vi "Test Test Case Status Correct When Collecting Method Result.vi"(8 "error in (no error)":errorcluster, 11 "Test Case In":refnum<class "Result Collector Tests.lvclass">) -> (0 "error out":errorcluster, 3 "Test Case Out":refnum<class "Result Collector Tests.lvclass">)   [LabVIEW 2020, in "Result Collector Tests.lvclass"]
uses:
  Result Collector Tests.lvclass
  C:/Program Files (x86)/National Instruments/LabVIEW 2020/vi.lib/Astemes/LUnit/Test Case.lvclass
  Framework/Result Collector/Result Collector.lvclass
  Result/Result.ctl
  Result/Status.ctl
  Result/Type.ctl
  Framework/Result Collector/Result Collector.lvclass/Result Collector.ctl
  <vilib>/Astemes/LUnit/Test Case.lvclass/Test Case.ctl
  7d523b10-b8d1-4baa-9334-5865d033fd32.vi
  Framework/Result Collector/Public/API/Collect Method Results.vi
  <vilib>/Astemes/LUnit/Palette/Pass.vi
  <vilib>/Astemes/LUnit/Palette/Fail.vi
  <vilib>/Astemes/LUnit/Compare Variants.vi
  <vilib>/Astemes/LUnit/Describe Comparison.vi
  <vilib>/Astemes/LUnit/Set Assertion Type.vi
  <vilib>/Astemes/LUnit/Add test result.vi
  <vilib>/Astemes/LUnit/Variant to string.vi
  <vilib>/Astemes/LUnit/LUnit Record Assertion Result.vi
  <vilib>/Astemes/LUnit/LUnit Aggregate Assertion Results.vi
  <vilib>/Astemes/LUnit/Method Result/LUnit Merge Status.vi
  <vilib>/Astemes/LUnit/LUnit Concatenate result strings.vi
  <vilib>/Utility/Data Type/Get Type Information.vi
  <vilib>/Utility/LVClass/Get LV Class Name.vi
  Result/Result.lvlib
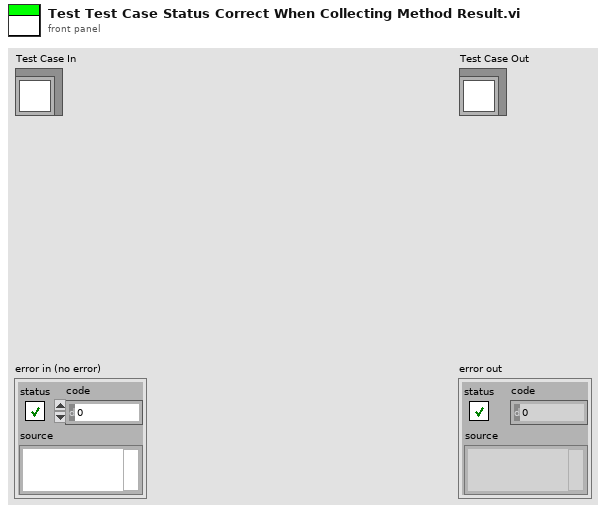
[diagram p1: front panel]
types:
  T1 = typedef "Result.lvlib/Status.ctl" = enum16{"Pass", "Fail", "Error", "Skipped", "Setup Error", "Broken", "Teardown Error"}
  T2 = typedef "Result.lvlib/Result.ctl" = cluster{"Case":string, "Method":string, "Message":string, "Description":string, "Status":T1, "Result Type":T3, "Execution Time":dbl}
  T3 = typedef "Result.lvlib/Type.ctl" = enum16{"Assertion", "Method", "Case", "Suite"}
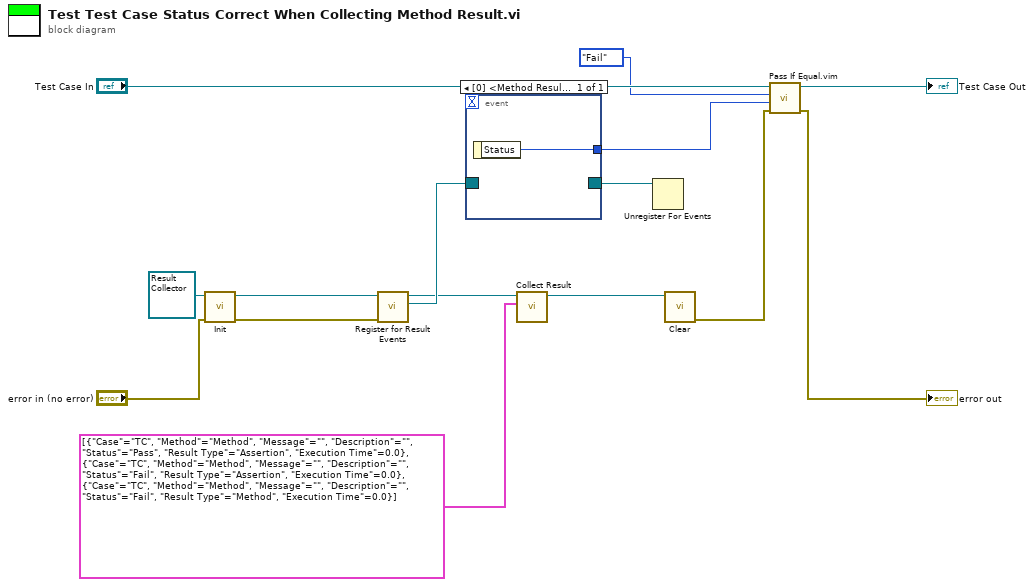
[diagram p0: block diagram]
diagram:
  n1 = call-dynamic "Init.vi"("error in (no error)"="error in (no error)", "Report Generator In"=refnum<class "Result Collector.lvclass"> refnum) -> ("error out"=w11:errorcluster, "Report Generator Out"=w12:refnum<class "Result Collector.lvclass">)  [unwired: 8 in]
  n2 = call "Register for Result Events.vi"("error in (no error)"=w11, "Result Collector In"=w12) -> ("Result Events"=w9:refnum<event-registration>, "Result Collector Out"=w7:refnum<class "Result Collector.lvclass">)  [unwired: 7 in, 1 out]
  n3 = event shown="[0] <Method Result>: User Event" {
    selector: w9 -> [_]
    dyn-events: [_] -> w8
    timeout: _ -> [_]
    tunnel: [w16] -> w4
    event User Event {
      n4 = event-data() -> ("Status"=w16:T1)  [unwired: 1 in]
    }
  }
  n5 = call "Collect Result.vi"("Results"=T2[] [{"Case"="TC", "Method"="Method", "Message"="", "Description"="", "Status"=enum."Pass", "Result Type"=enum."Assertion", "Execution Time"=0.0}, {"Case"="TC", "Method"="Method", "Message"="", "Description"="", "Status"=enum."Fail", "Result Type"=enum."Assertion", "Execution Time"=0.0}, {"Case"="TC", "Method"="Method", "Message"="", "Description"="", "Status"=enum."Fail", "Result Type"=enum."Method", "Execution Time"=0.0}], "Report Generator In"=w7) -> ("Report Generator Out"=w6:refnum<class "Result Collector.lvclass">)  [unwired: 9 in]
  n6 = Unregister For Events(event registration refnum=w8) -> ()  [unwired: 1 in, 1 out]
  n7 = call-dynamic "Clear.vi"("Report Generator In"=w6) -> ("error out"=w3:errorcluster)  [unwired: 9 in, 1 out]
  n8 = call "Pass If Equal.vim"("error in (no error)"=w3, "Actual"=w4, "Expected"=Status."Fail" ("Status"), "LUnit Test Case In"="Test Case In") -> ("error out"=→"error out":errorcluster, "LUnit Test Case Out"=→"Test Case Out":refnum<class "Result Collector Tests.lvclass">)  [unwired: 6 in]
